vi "generic query.vi"() -> ()   [LabVIEW 2013, in "Universal Power Meter.lvlib"]
uses:
  Universal Power Meter.lvlib
  <instrlib>/Yokogawa WT200 Series/Yokogawa WT200 Series.lvlib
panel:
  out "substring":string
  out "Start":string="1001001001010"
  out "RES!":string="1001001001000"
  out "BINARY":string
  in  "Response?":bool
  out "error out":errorcluster
  in  "write buffer":string
  in  "VISA resource name":refnum<visa-resource-name>
  out "read buffer":string
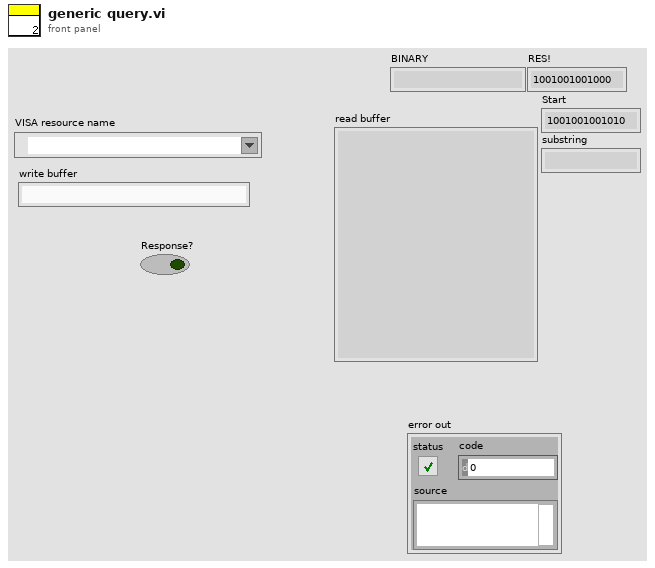
[diagram p1: front panel]
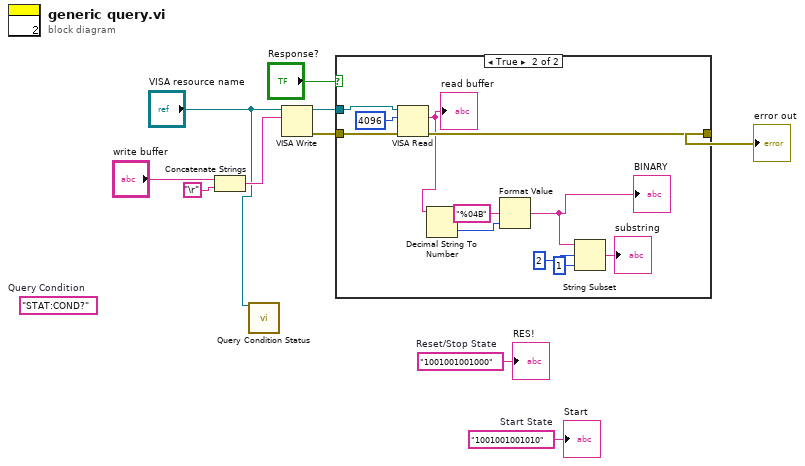
[diagram p0: block diagram]
diagram:
  (unwired) "STAT:COND?"  # Query Condition
  w2 = "1001001001010"  # Start State
  w3 = "1001001001000"  # Reset/Stop State
  n1 = Concatenate Strings("write buffer", "\r") -> (w4:string)
  n2 = call <instrlib>:"Query Condition Status.vi"("VISA resource name"="VISA resource name") -> ()  [unwired: 12 in, 3 out]
  n3 = VISA Write(VISA resource name="VISA resource name", write buffer=w4) -> (VISA resource name out=w10:refnum<visa-resource-name>, error out=w9:errorcluster)  [unwired: 1 in, 1 out]
  n4 = case shown="True" "Response?" {
    tunnel: w10 -> [_ w22]
    tunnel: w9 -> [w11 w21]
    tunnel: [w11 w19] -> w8
    frame False {
    }
    frame True {
      n5 = VISA Read(VISA resource name=w22, byte count=u32 4096, error in (no error)=w21) -> (read buffer=w17:string, error out=w19:errorcluster)  [unwired: 2 out]
      "read buffer" <- w17
      n6 = Decimal String To Number(string=w17) -> (number=w16:i32)  [unwired: 2 in, 1 out]
      n7 = Format Value(format string="%04B", value (0)=w16) -> (output string=w15:string)  [unwired: 1 in]
      "BINARY" <- w15
      n8 = String Subset(string=w15, offset (0)=2, length (rest)=1 ("length (rest)")) -> (substring=→"substring":string)
    }
  }
  "error out" <- w8
  "RES!" <- w3
  "Start" <- w2
